vi "Get Summary.vi"(8 "error in (no error)":errorcluster, 10 "Item":string, 11 "Result Model In":refnum<class "Result Model.lvclass">) -> (0 "error out":errorcluster, 2 "Summary":string)   [LabVIEW 2020, in "Result Model.lvclass"]
uses:
  Result Model.lvclass
  Result Model.lvclass/Result Model.ctl
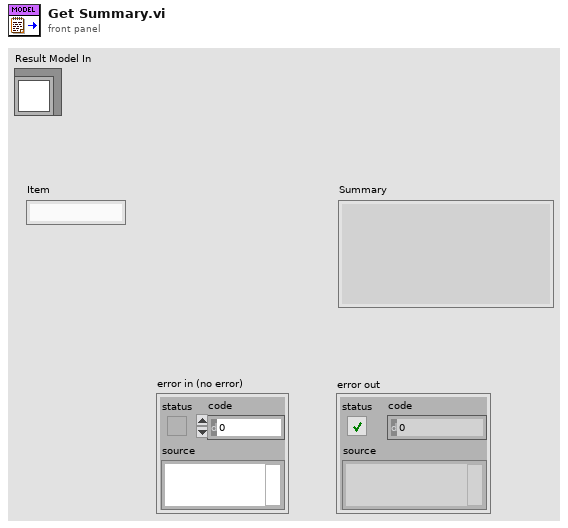
[diagram p1: front panel]
types:
  T1 = typedef "Result.lvlib/Status.ctl" = enum16{"", "Passed", "Failed", "Error", "Skipped", "Setup Error", "Broken", "Teardown Error"}
  T2 = typedef "Result.lvlib/Type.ctl" = enum16{"Test Case", "Test Suite", "Test Run", "Pass", "Fail", "Skip", "Pass if", "Fail if", "Pass if Error", "Fail if Error", "Pass if Equal", "Fail if Equal"}
  T3 = map{string, cluster{"Result Type":T2, "Status":T1, "Message":string, "Description":string}[]}
  T4 = cluster{"Result Type":T2, "Status":T1, "Message":string, "Description":string}[]
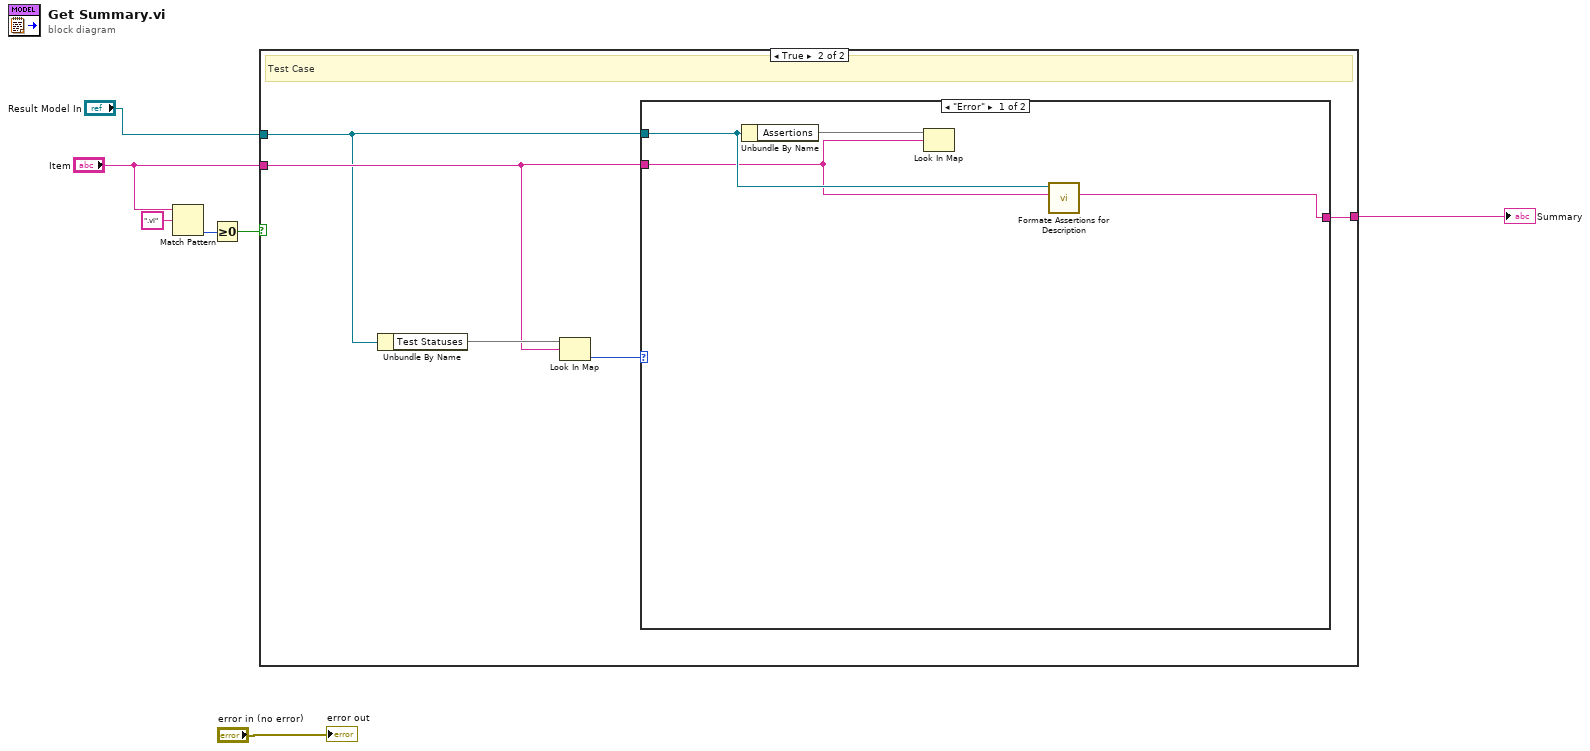
[diagram p0: block diagram]
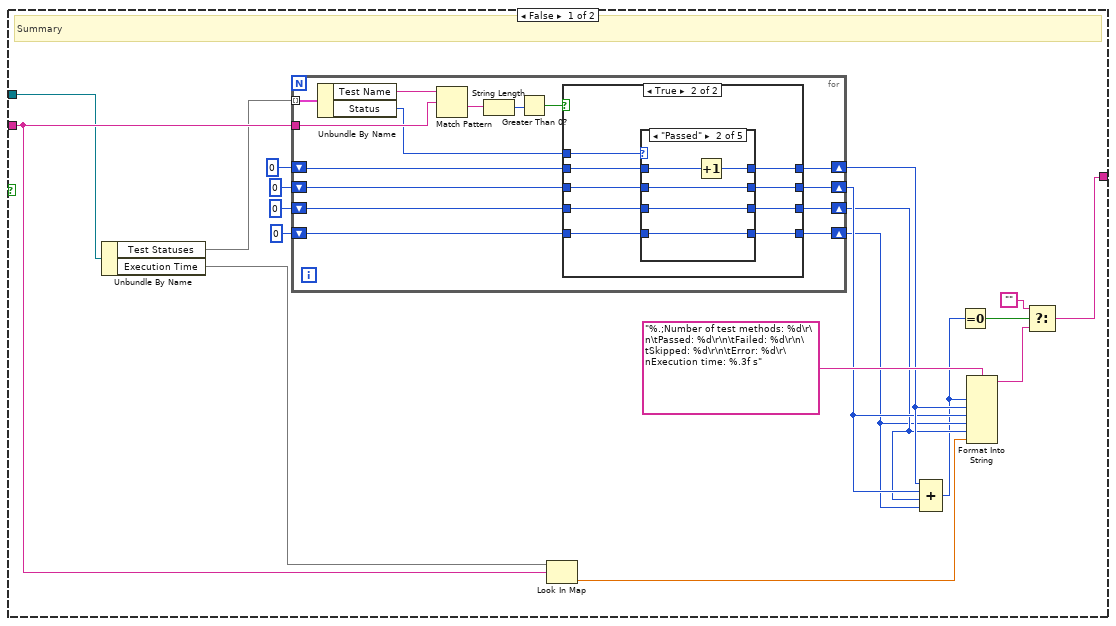
[diagram p2: hidden frame]
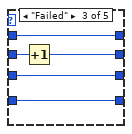
[diagram p5: hidden frame]
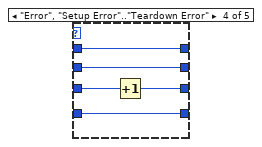
[diagram p6: hidden frame]
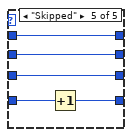
[diagram p7: hidden frame]
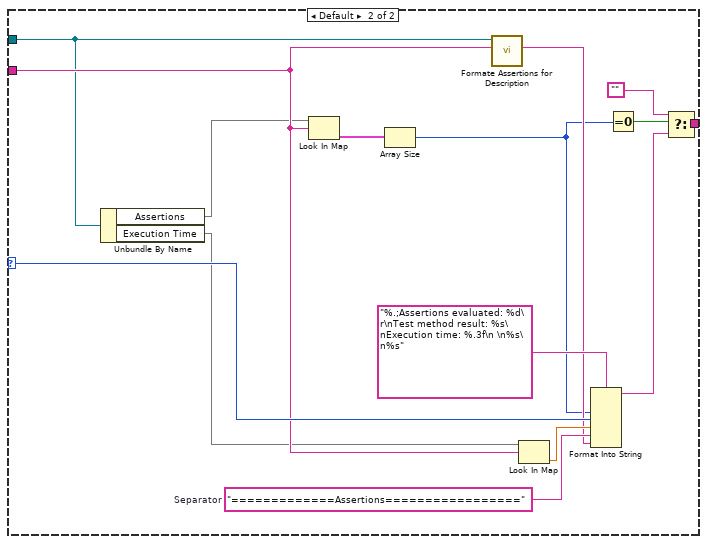
[diagram p8: hidden frame]
diagram:
  n1 = Match Pattern(string="Item", regular expression=".vi") -> (offset past match=w6:i32)  [unwired: 1 in, 3 out]
  n2 = Greater Or Equal To 0?(x=w6) -> (x >= 0?=w5:bool)
  n3 = case shown="True" w5 {
    tunnel: "Item" -> [w24 w80]
    tunnel: [w12 w82] -> w3
    tunnel: "Result Model In" -> [w8 w79]
    frame False {
      # "Summary"
      n4 = Unbundle By Name(w8) -> ("Test Statuses"=w10:map{string, T1}, "Execution Time"=w9:map{string, dbl})
      n5 = for {
        tunnel: w10 -> [w41] mode=indexing
        tunnel: w24 -> [w39]
        shift-right: [w35] -> w22
        shift-left: 0 ("value") -> [w37]
        shift-right: [w33] -> w20
        shift-left: 0 ("value") -> [w34]
        shift-right: [w31] -> w18
        shift-left: 0 ("value") -> [w32]
        shift-right: [w30] -> w16
        shift-left: 0 ("value") -> [w29]
        n6 = Unbundle By Name(w41) -> ("Test Name"=w40:string, "Status"=w38:T1)
        n7 = Match Pattern(string=w40, regular expression=w39) -> (after substring=w28:string)  [unwired: 1 in, 3 out]
        n8 = String Length(string=w28) -> (length=w27:i32)
        n9 = Greater Than 0?(x=w27) -> (x > 0?=w36:bool)
        n10 = case shown="True" w36 {
          tunnel: w38 -> [_ w54]
          tunnel: w37 -> [w45 w53]
          tunnel: [w45 w52] -> w35
          tunnel: w34 -> [w44 w51]
          tunnel: [w44 w50] -> w33
          tunnel: w32 -> [w42 w49]
          tunnel: [w42 w48] -> w31
          tunnel: [w43 w47] -> w30
          tunnel: w29 -> [w43 w46]
          frame False {
          }
          frame True {
            n11 = case shown="\"Passed\"" w54 {
              tunnel: w53 -> [w58 w63 w68 w72 w78]
              tunnel: [w58 w62 w68 w72 w78] -> w52
              tunnel: w51 -> [w57 w61 w67 w73 w77]
              tunnel: [w57 w61 w66 w73 w77] -> w50
              tunnel: w49 -> [w56 w60 w65 w71 w76]
              tunnel: [w56 w60 w65 w70 w76] -> w48
              tunnel: [w55 w59 w64 w69 w74] -> w47
              tunnel: w46 -> [w55 w59 w64 w69 w75]
              frame "" {
              }
              frame "Passed" {
                n12 = Increment(x=w63) -> (x+1=w62:i32)
              }
              frame "Failed" {
                n13 = Increment(x=w67) -> (x+1=w66:i32)
              }
              frame "Error", "Setup Error".."Teardown Error" {
                n14 = Increment(x=w71) -> (x+1=w70:i32)
              }
              frame "Skipped" {
                n15 = Increment(x=w75) -> (x+1=w74:i32)
              }
            }
          }
        }
      }
      n16 = Look In Map(map=w9, key=w24) -> (value=w25:dbl)  [unwired: 1 in, 1 out]
      n17 = Compound Arithmetic op=ADD(w22, w20, w18, w16) -> (w15:i32)
      n18 = Equal To 0?(x=w15) -> (x = 0?=w14:bool)
      n19 = Format Into String(format string="%.;Number of test methods: %d\r\n\tPassed: %d\r\n\tFailed: %d\r\n\tSkipped: %d\r\n\tError: %d\r\nExecution time: %.3f s", w15, w22, w20, w16, w18, w25) -> (resulting string=w13:string)  [unwired: 2 in, 1 out]
      n20 = Select(t="", s=w14, f=w13) -> (s? t:f=w12:string)
    }
    frame True {
      # "Test Case"
      n21 = Unbundle By Name(w79) -> ("Test Statuses"=w81:map{string, T1})
      n22 = Look In Map(map=w81, key=w80) -> (value=w83:T1)  [unwired: 1 in, 1 out]
      n23 = case shown="\"Error\"" w83 {
        selector: w83 -> [_ w99]
        tunnel: [w84 w93] -> w82
        tunnel: w80 -> [w85 w91]
        tunnel: w79 -> [w86 w90]
        frame "Error" {
          n24 = Unbundle By Name(w86) -> ("Assertions"=w87:T3)
          n25 = Look In Map(map=w87, key=w85) -> ()  [unwired: 1 in, 2 out]
          n26 = call "Formate Assertions for Description.vi"("Item"=w85, "Result Model In"=w86) -> ("Assertions Description"=w84:string)  [unwired: 9 in]
        }
        frame Default {
          w101 = "=============Assertions================="  # Separator
          n27 = Unbundle By Name(w90) -> ("Assertions"=w88:T3, "Execution Time"=w89:map{string, dbl})
          n28 = Look In Map(map=w88, key=w91) -> (value=w97:T4)  [unwired: 1 in, 1 out]
          n29 = Array Size(array=w97) -> (size(s)=w96:i32)
          n30 = call "Formate Assertions for Description.vi"("Item"=w91, "Result Model In"=w90) -> ("Assertions Description"=w98:string)  [unwired: 9 in]
          n31 = Look In Map(map=w89, key=w91) -> (value=w100:dbl)  [unwired: 1 in, 1 out]
          n32 = Format Into String(format string="%.;Assertions evaluated: %d\r\nTest method result: %s\nExecution time: %.3f\n \n%s\n%s", w96, w99, w100, w101, w98) -> (resulting string=w94:string)  [unwired: 2 in, 1 out]
          n33 = Equal To 0?(x=w96) -> (x = 0?=w95:bool)
          n34 = Select(t="", s=w95, f=w94) -> (s? t:f=w93:string)
        }
      }
    }
  }
  "Summary" <- w3
  "error out" <- "error in (no error)"
